vi "Logger.ReadResultFile.vi"(8 "error in":errorcluster, 11 "ResultFilePath":path) -> (0 "error out":errorcluster, 1 "ResultValues":dbl[](array[numeric]), 2 "ResultValues":string[](array[string]), 3 "text":string)   [LabVIEW 2016]
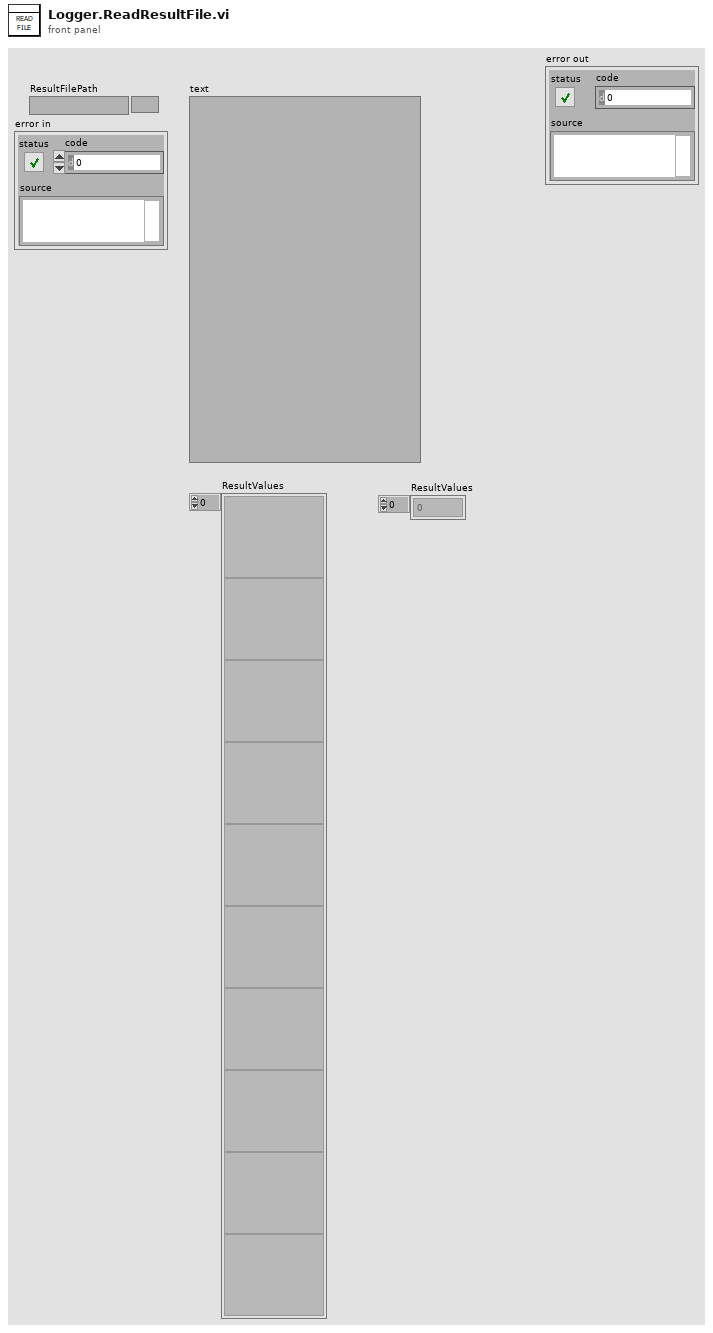
[diagram p1: front panel]
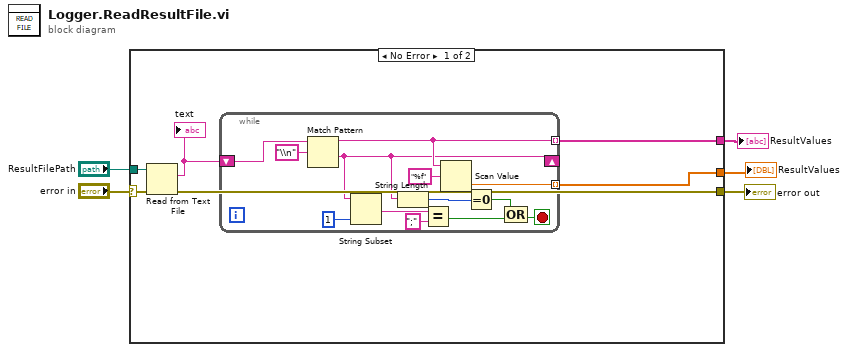
[diagram p0: block diagram]
diagram:
  n1 = case shown="No Error" "error in" {
    selector: "error in" -> [w8 w25]
    tunnel: "ResultFilePath" -> [w10 _]
    tunnel: [w9 w25] -> w4
    tunnel: [w7 _] -> w2
    tunnel: [w6 _] -> w1
    frame No Error {
      n2 = Read from Text File(file (use dialog)=w10, error in=w8) -> (text=w11:string, error out=w9:errorcluster)  [unwired: 2 in, 2 out]
      "text" <- w11
      n3 = while {
        tunnel: [w21] -> w7 mode=indexing
        shift-right: [w14] -> _
        shift-left: w11 -> [w24]
        tunnel: [w19] -> w6 mode=indexing
        stop <- w15 stop-if-true
        n4 = Match Pattern(string=w24, regular expression="\\n") -> (before substring=w21:string, after substring=w14:string)  [unwired: 1 in, 2 out]
        n5 = String Subset(string=w14, length (rest)=1 ("length (rest)")) -> (substring=w12:string)  [unwired: 1 in]
        n6 = String Length(string=w14) -> (length=w23:i32)
        n7 = Equal?(x=w12, y=";") -> (x = y?=w16:bool)
        n8 = Scan Value(string=w21, format string="%f") -> (value=w19:dbl)  [unwired: 1 in, 1 out]
        n9 = Equal To 0?(x=w23) -> (x = 0?=w17:bool)
        n10 = Compound Arithmetic op=OR(w17, w16) -> (w15:bool)
      }
    }
    frame Error {
    }
  }
  "error out" <- w4
  "ResultValues" <- w1
  "ResultValues" <- w2
